vi "AKD Move.vi"(0 "TCP Refnum in":refnum<k5>, 5 "Motion Task parameters":T1={"Target position (mm)"=0.0, "Target velocity (mm/s)"=0.0, "Motion type"=enum."Rel", "Target acc (mm/s^2)"=1000.0, "Target dec (mm/s^2)"=1000.0}, 11 "error in 2":errorcluster) -> (4 "TCP Refnum out":refnum<k5>, 15 "error out 2":errorcluster)   [LabVIEW 2019]
uses:
  MODBUS/NI Modbus.llb/MB Ethernet Master Query Write Multiple Registers (poly).vi
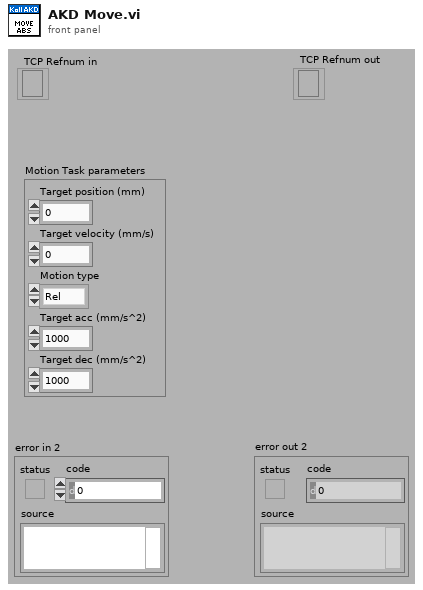
[diagram p1: front panel]
types:
  T1 = cluster{"Target position (mm)":sgl, "Target velocity (mm/s)":sgl, "Motion type":enum16{"Rel", "Abs"}, "Target acc (mm/s^2)":sgl, "Target dec (mm/s^2)":sgl}
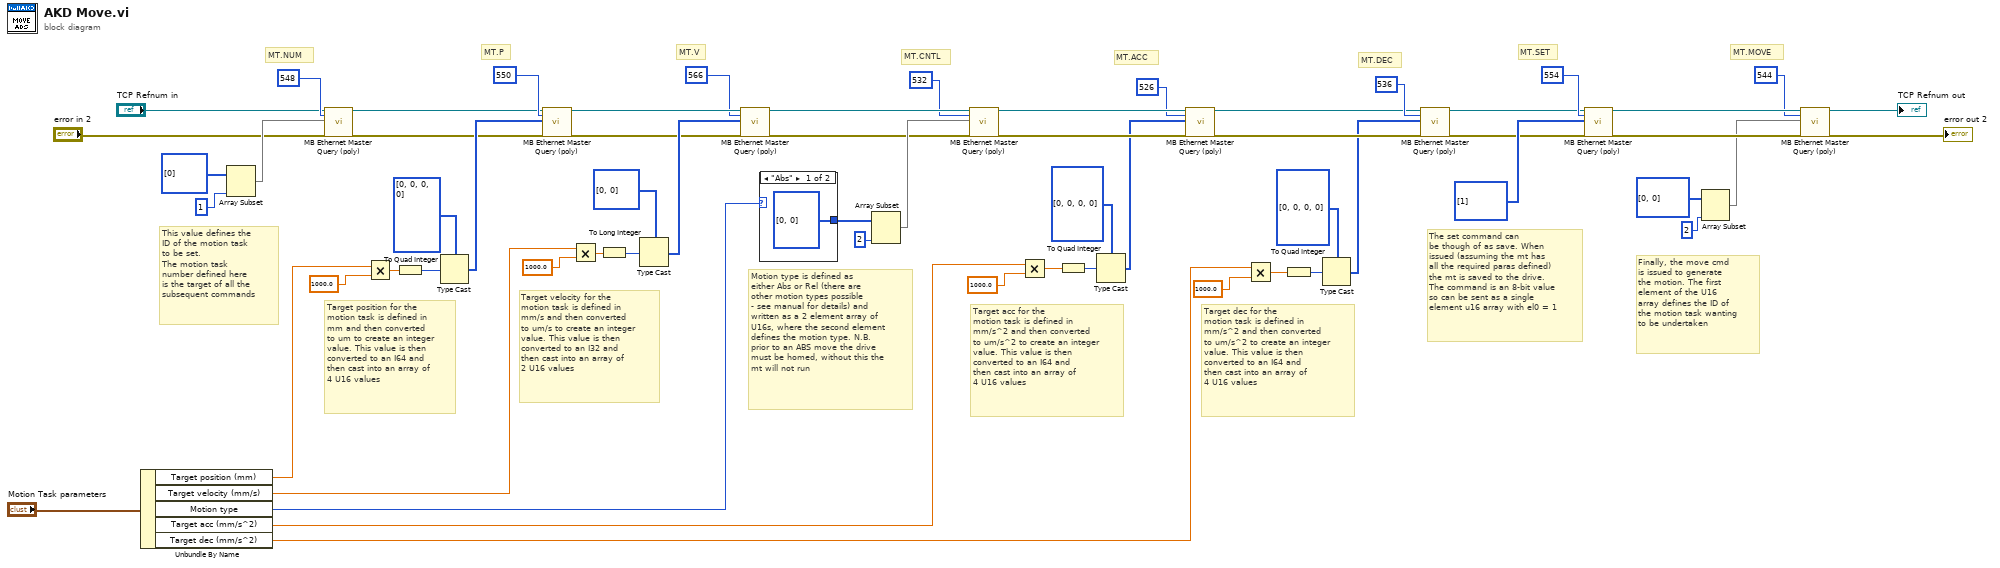
[diagram p0: block diagram]
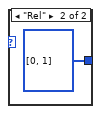
[diagram p2: hidden frame]
diagram:
  # "Finally, the move cmd\nis issued to generate\nthe motion. The first\nelement of the U16\narray defines the ID of\nthe motion task wanting\nto be undertaken"
  # "The set command can\nbe though of as save. When\nissued (assuming the mt has \nall the required paras defined)\nthe mt is saved to the drive.\nThe command is an 8-bit value\nso can be sent as a single\nelement u16 array with el0 = 1"
  # "Target dec for the\nmotion task is defined in\nmm/s^2 and then converted\nto um/s^2 to create an integer\nvalue. This value is then\nconverted to an I64 and\nthen cast into an array of \n4 U16 values"
  # "Target acc for the\nmotion task is defined in\nmm/s^2 and then converted\nto um/s^2 to create an integer\nvalue. This value is then\nconverted to an I64 and\nthen cast into an array of \n4 U16 values"
  # "Motion type is defined as\neither Abs or Rel (there are\nother motion types possible\n- see manual for details) and\nwritten as a 2 element array of\nU16s, where the second element\ndefines the motion type. N.B.\nprior to an ABS move the drive\nmust be homed, without this the\nmt will not run"
  # "Target velocity for the\nmotion task is defined in\nmm/s and then converted\nto um/s to create an integer\nvalue. This value is then\nconverted to an I32 and\nthen cast into an array of \n2 U16 values"
  # "Target position for the\nmotion task is defined in\nmm and then converted\nto um to create an integer\nvalue. This value is then\nconverted to an I64 and\nthen cast into an array of \n4 U16 values"
  # "This value defines the \nID of the motion task\nto be set.\nThe motion task\nnumber defined here\nis the target of all the \nsubsequent commands"
  # "MT.MOVE"
  # "MT.DEC"
  # "MT.ACC"
  # "MT.SET"
  # "MT.CNTL"
  # "MT.V"
  # "MT.P"
  # "MT.NUM"
  n1 = Unbundle By Name("Motion Task parameters") -> ("Target position (mm)"=w5:sgl, "Target velocity (mm/s)"=w4:sgl, "Motion type"=w3:enum16{"Rel", "Abs"}, "Target acc (mm/s^2)"=w2:sgl, "Target dec (mm/s^2)"=w1:sgl)
  n2 = Array Subset(array=u16[] [0], length=1) -> (w59:u16[])  [unwired: 1 in]
  n3 = call-poly "MB Ethernet Master Query (poly).vi"("TCP Connection Refnum in"="TCP Refnum in", "Starting Address"=u16 548, "Registers"=w59, "error in"="error in 2") -> ("TCP Connection Refnum (dup)"=w25:refnum<k5>, "error out"=w24:errorcluster)  [unwired: 13 in, 1 out]
  n4 = Multiply(x=w5, y=sgl 1000.0) -> (x*y=w17:sgl)
  n5 = To Quad Integer(1:w17) -> (0:w15:i64)
  n6 = Type Cast(type=u16[] [0, 0, 0, 0], x=w15) -> (*(type *) &x=w56:u16[])
  n7 = call-poly "MB Ethernet Master Query (poly).vi"("TCP Connection Refnum in"=w25, "Starting Address"=u16 550, "Registers"=w56, "error in"=w24) -> ("TCP Connection Refnum (dup)"=w53:refnum<k5>, "error out"=w45:errorcluster)  [unwired: 13 in, 1 out]
  n8 = Multiply(x=w4, y=sgl 1000.0) -> (x*y=w13:sgl)
  n9 = To Long Integer(number=w13) -> (32bit integer=w14:i32)
  n10 = Type Cast(type=u16[] [0, 0], x=w14) -> (*(type *) &x=w54:u16[])
  n11 = call-poly "MB Ethernet Master Query (poly).vi"("TCP Connection Refnum in"=w53, "Starting Address"=u16 566, "Registers"=w54, "error in"=w45) -> ("TCP Connection Refnum (dup)"=w51:refnum<k5>, "error out"=w44:errorcluster)  [unwired: 13 in, 1 out]
  n12 = case shown="\"Abs\"" w3 {
    tunnel: [u16[] [0, 0] u16[] [0, 1]] -> w46
    frame "Abs" {
    }
    frame "Rel" {
    }
  }
  n13 = Array Subset(array=w46, length=2) -> (w48:u16[])  [unwired: 1 in]
  n14 = call-poly "MB Ethernet Master Query (poly).vi"("TCP Connection Refnum in"=w51, "Starting Address"=u16 532, "Registers"=w48, "error in"=w44) -> ("TCP Connection Refnum (dup)"=w42:refnum<k5>, "error out"=w37:errorcluster)  [unwired: 13 in, 1 out]
  n15 = Multiply(x=w2, y=sgl 1000.0) -> (x*y=w33:sgl)
  n16 = To Quad Integer(1:w33) -> (0:w32:i64)
  n17 = Type Cast(type=u16[] [0, 0, 0, 0], x=w32) -> (*(type *) &x=w36:u16[])
  n18 = call-poly "MB Ethernet Master Query (poly).vi"("TCP Connection Refnum in"=w42, "Starting Address"=u16 526, "Registers"=w36, "error in"=w37) -> ("TCP Connection Refnum (dup)"=w35:refnum<k5>, "error out"=w38:errorcluster)  [unwired: 13 in, 1 out]
  n19 = Multiply(x=w1, y=sgl 1000.0) -> (x*y=w10:sgl)
  n20 = To Quad Integer(1:w10) -> (0:w11:i64)
  n21 = Type Cast(type=u16[] [0, 0, 0, 0], x=w11) -> (*(type *) &x=w7:u16[])
  n22 = call-poly "MB Ethernet Master Query (poly).vi"("TCP Connection Refnum in"=w35, "Starting Address"=u16 536, "Registers"=w7, "error in"=w38) -> ("TCP Connection Refnum (dup)"=w27:refnum<k5>, "error out"=w26:errorcluster)  [unwired: 13 in, 1 out]
  n23 = call-poly "MB Ethernet Master Query (poly).vi"("TCP Connection Refnum in"=w27, "Starting Address"=u16 554, "Registers"=u16[] [1], "error in"=w26) -> ("TCP Connection Refnum (dup)"=w28:refnum<k5>, "error out"=w29:errorcluster)  [unwired: 13 in, 1 out]
  n24 = Array Subset(array=u16[] [0, 0], length=2) -> (w21:u16[])  [unwired: 1 in]
  n25 = call-poly "MB Ethernet Master Query (poly).vi"("TCP Connection Refnum in"=w28, "Starting Address"=u16 544, "Registers"=w21, "error in"=w29) -> ("TCP Connection Refnum (dup)"=→"TCP Refnum out":refnum<k5>, "error out"=→"error out 2":errorcluster)  [unwired: 13 in, 1 out]
